vi "Actor Core.vi"(8 "error in":errorcluster, 11 "Simulated ParameterDevice in":refnum<class "Simulated ParameterDevice.lvclass">) -> (0 "error out":errorcluster, 3 "Actor out":refnum<class "Actor.lvclass">)   [LabVIEW 2014, in "Simulated ParameterDevice.lvclass"]
doc: "(<B>Filename</B>: Actor Framework.lvlib:Actor.lvclass:Actor Core.vi)\n\nReceives messages to the actor, reacts to them, and initiates any error handling that may shut the actor down.\n\nDescendant classes may override this VI to append parallel tasks for the actor to complete while it handles messages. Overrides use the Call Parent Method node."
uses:
  Simulated ParameterDevice.lvclass
  <vilib>/ActorFramework/Actor/Actor.lvclass
  <vilib>/ActorFramework/Actor/Actor.lvclass/Actor.ctl
  <vilib>/ActorFramework/Message Enqueuer/Message Enqueuer.lvclass/Message Enqueuer.ctl
  <vilib>/ActorFramework/Message Enqueuer/Init from Existing Queue.vi
  <vilib>/ActorFramework/Message Enqueuer/Message Enqueuer.lvclass
  Framework/Hardware/ParameterDevice/ParameterDevice.lvclass
  Framework/Interfaces/Viewable Actor/Viewable Actor.lvclass
  Framework/Interfaces/Observable Actor/Observable Actor.lvclass
panel:
  out "Stop":bool=TRUE
  out "Current value":dbl
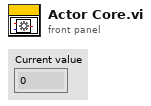
[diagram p1: front panel]
types:
  T1 = typedef "Observable Actor.lvlib/Observable Actor.lvclass/Observer.ctl" = refnum<queue>
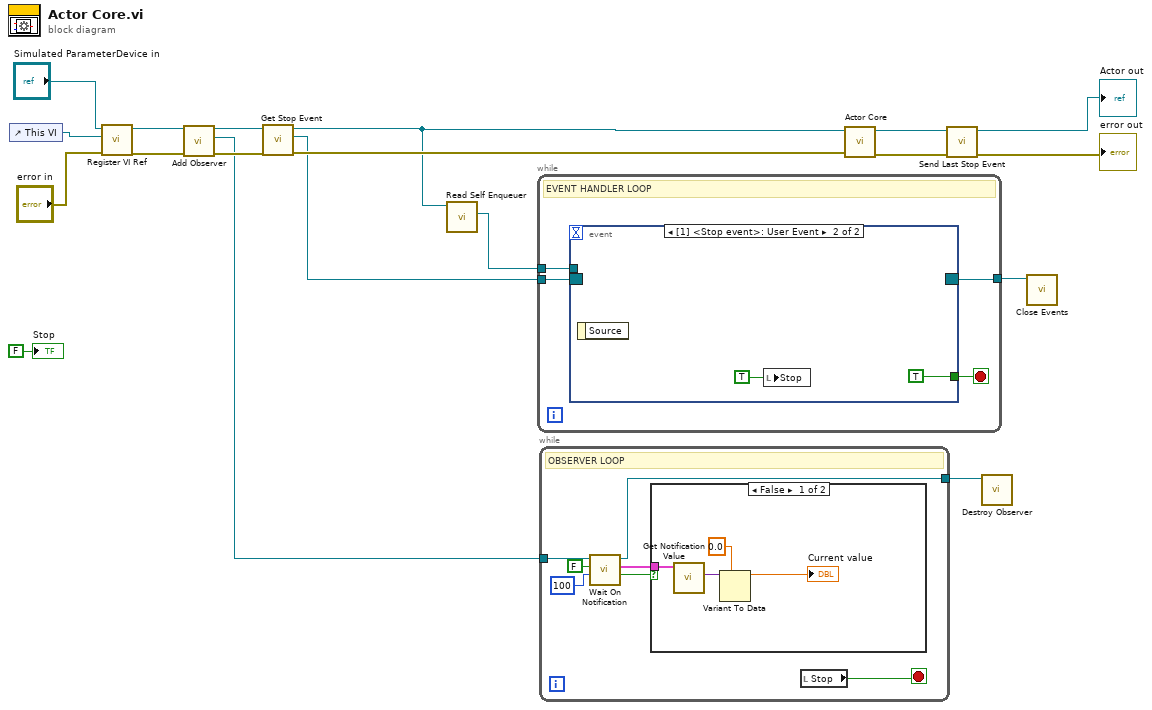
[diagram p0: block diagram]
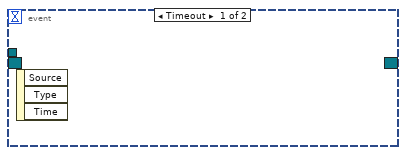
[diagram p3: hidden frame]
diagram:
  n1 = control-ref of="This VI"() -> (w17:refnum<vi>)
  n2 = call "Register VI Ref.vi"("error in (no error)"="error in", "VI ref"=w17, "Viewable Actor in"="Simulated ParameterDevice in") -> ("error out"=w2:errorcluster, "Viewable Actor out"=w1:refnum<class "Simulated ParameterDevice.lvclass">)  [unwired: 7 in]
  n3 = call-dynamic "Add Observer.vi"("error in (no error)"=w2, "Observable Actor in"=w1) -> ("error out"=w16:errorcluster, "new observer"=w14:T1, "Observable Actor out"=w13:refnum<class "Simulated ParameterDevice.lvclass">)  [unwired: 7 in]
  n4 = call-dynamic "Get Stop Event.vi"("error in (no error)"=w16, "Observable Actor in"=w13) -> ("error out"=w12:errorcluster, "Events"=w11:refnum<event-registration>, "Observable Actor out"=w6:refnum<class "Simulated ParameterDevice.lvclass">)  [unwired: 7 in]
  n5 = call <vilib>:"Read Self Enqueuer.vi"("Actor"=w6) -> ("Self Enqueuer"=w15:refnum<class "Message Enqueuer.lvclass">)  [unwired: 10 in]
  n6 = while {
    tunnel: w11 -> [w23]
    tunnel: w15 -> [w22]
    tunnel: [w21] -> w10
    stop <- w20 stop-if-true
    # "EVENT HANDLER LOOP"
    n7 = event shown="[1] <Stop event>: User Event" {
      selector: w23 -> [_ _]
      dyn-events: [_ _] -> w21
      timeout: _ -> [_ _]
      tunnel: w22 -> [_ _]
      tunnel: [_ TRUE] -> w20
      event Timeout {
        n8 = event-data() -> ()  [unwired: 1 in, 3 out]
      }
      event User Event {
        n9 = event-data() -> ()  [unwired: 1 in, 1 out]
        n10 = local write "Stop"(TRUE ("Stop")) -> ()
      }
    }
  }
  n11 = while {
    tunnel: w14 -> [w27]
    tunnel: [w26] -> w7
    stop <- w32 stop-if-true
    # "OBSERVER LOOP"
    n12 = call "Wait On Notification.vi"("timeout in ms (-1)"=100, "ignore previous (F)"=FALSE, "observer in"=w27) -> ("timed out?"=w28:bool, "notification"=w29:cluster{"value":variant, "name":string}, "observer out"=w26:T1)  [unwired: 5 in, 1 out]
    n13 = case shown="False" w28 {
      tunnel: w29 -> [w36 _]
      frame False {
        n14 = call "Get Notification Value.vi"("notification in"=w36) -> ("data"=w35:variant)  [unwired: 7 in, 1 out]
        n15 = Variant To Data(type=0.0 ("Current value"), Variant=w35) -> (data=→"Current value":dbl)  [unwired: 1 in, 1 out]
      }
      frame True {
      }
    }
    n16 = local read "Stop"() -> (w32:bool)
  }
  n17 = call-parent "Actor Core.vi"("error in"=w12, "Actor in"=w6) -> ("error out"=w8:errorcluster, "Actor out"=w9:refnum<class "Actor.lvclass">)  [unwired: 8 in]
  n18 = call "Send Last Stop Event.vi"("error in (no error)"=w8, "Actor in"=w9) -> ("error out"=→"error out":errorcluster, "Actor  out"=→"Actor out":refnum<class "Actor.lvclass">)  [unwired: 8 in]
  n19 = call "Destroy Observer.vi"("observer in"=w7) -> ()  [unwired: 11 in]
  n20 = call "Close Events.vi"("events"=w10) -> ()  [unwired: 11 in]
  "Stop" <- FALSE ("Stop")
